vi "Cleanup.vi"(8 "error in (no error)":errorcluster, 11 "TCPMessaging in":refnum<class "TCPMessaging.lvclass">) -> (0 "error out":errorcluster)   [LabVIEW 2020, in "Vecto.lvlib" / "TCPMessaging.lvclass"]
uses:
  TCPMessaging.lvclass
  TCPMessaging.lvclass/TCPMessaging.ctl
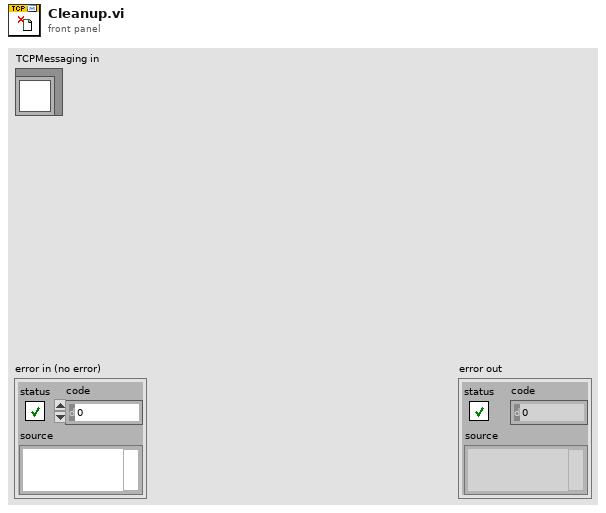
[diagram p1: front panel]
types:
  T1 = typedef "Vecto.lvlib/TCPMessaging.lvclass/TCP Mode.ctl" = enum16{"Client", "Server"}
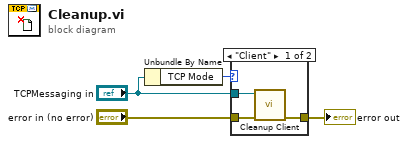
[diagram p0: block diagram]
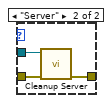
[diagram p2: hidden frame]
diagram:
  n1 = Unbundle By Name("TCPMessaging in") -> ("TCP Mode"=w3:T1)
  n2 = case shown="\"Client\"" w3 {
    tunnel: "error in (no error)" -> [w7 w10]
    tunnel: "TCPMessaging in" -> [w6 w9]
    tunnel: [w5 w8] -> w1
    frame "Client" {
      n3 = call "Cleanup Client.vi"("error in (no error)"=w7, "TCPMessaging in"=w6) -> ("error out"=w5:errorcluster)  [unwired: 9 in]
    }
    frame "Server" {
      n4 = call "Cleanup Server.vi"("error in (no error)"=w10, "TCPMessaging in"=w9) -> ("error out"=w8:errorcluster)  [unwired: 9 in]
    }
  }
  "error out" <- w1
